vi "Process - Set Status.vi"(0 "Module Data In":T2, 5 "Status":T1, 11 "error in (no error)":errorcluster) -> (4 "Module Data Out":T2, 15 "error out":errorcluster)   [LabVIEW 2020, in "Template.lvlib"]
doc: "Sets the status of the current process the Module is going through"
uses:
  Template.lvlib
  Controls/Module - Data.ctl
  Modules.ctl
  Controls/Module - States.ctl
  Controls/Timing - Data.ctl
  Controls/Process - Element.ctl
  Controls/Process.ctl
  Controls/Process - Status.ctl
  Error Handler - Logger Module/Error Handler - Logger.lvlib
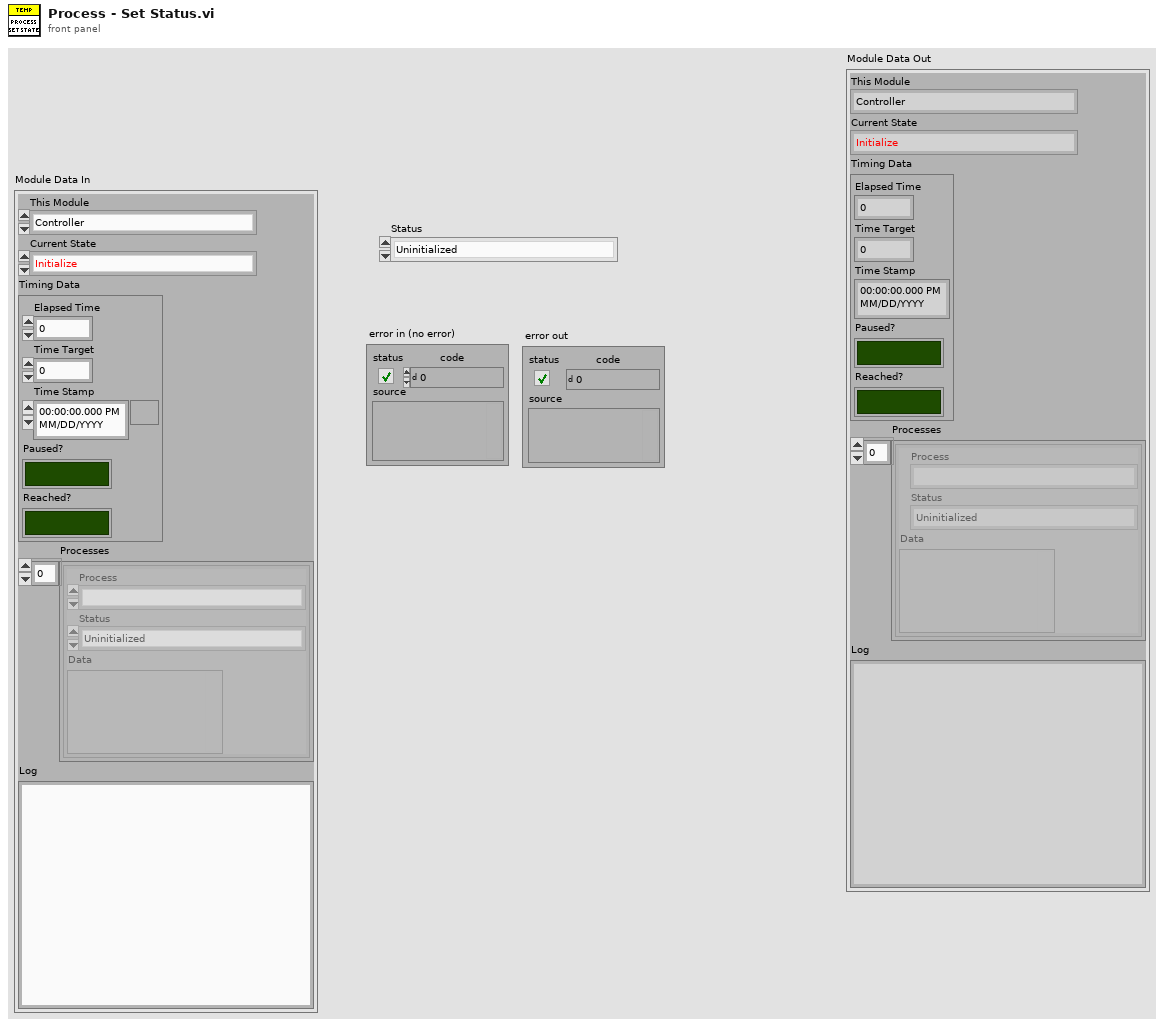
[diagram p1: front panel]
types:
  T1 = typedef "Template.lvlib/Process - Status.ctl" = enum16{"Uninitialized", "Busy"}
  T2 = typedef "Template.lvlib/Module - Data.ctl" = cluster{"This Module":T3, "Current State":T4, "Timing Data":T5, "Processes":T6[], "Log":string}
  T3 = typedef "Error Handler - Logger.lvlib/Modules.ctl" = enum16{"Controller", "Error Handler - Logger"}
  T4 = typedef "Template.lvlib/Module - States.ctl" = enum16{"Initialize", "Event ", "Send data", "FP Element: Update", "FP Element: Disable/Enable", "Timer: Setup", "Terminate", "---------------Template---------------"}
  T5 = typedef "Template.lvlib/Timing - Data.ctl" = cluster{"Elapsed Time":dbl, "Time Target":dbl, "Time Stamp":timestamp, "Paused?":bool, "Reached?":bool}
  T6 = typedef "Template.lvlib/Process - Element.ctl" = cluster{"Process":T7, "Status":T1, "Data":variant}
  T7 = typedef "Template.lvlib/Process.ctl" = enum16{""}
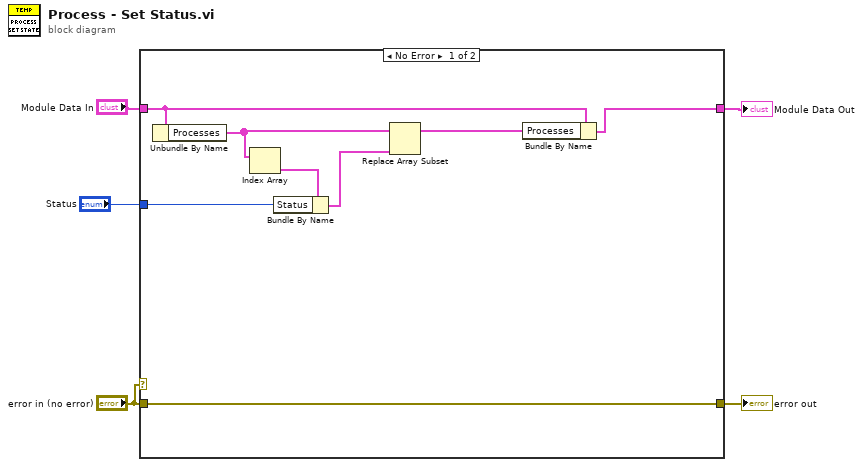
[diagram p0: block diagram]
diagram:
  n1 = case shown="No Error" "error in (no error)" {
    tunnel: [w7 w15] -> w5
    tunnel: "Module Data In" -> [w8 w15]
    tunnel: [w13 w14] -> w3
    tunnel: "error in (no error)" -> [w13 w14]
    tunnel: "Status" -> [w11 _]
    frame No Error {
      n2 = Unbundle By Name(w8) -> ("Processes"=w6:T6[])
      n3 = Index Array(array=w6) -> (element=w12:T6)  [unwired: 1 in]
      n4 = Bundle By Name(cluster=w12, "Status"=w11) -> (w10:T6)
      n5 = Replace Array Subset(array=w6, new element=w10) -> (w9:T6[])  [unwired: 1 in]
      n6 = Bundle By Name(cluster=w8, "Processes"=w9) -> (w7:T2)
    }
    frame Error {
    }
  }
  "error out" <- w3
  "Module Data Out" <- w5
